vi "Close Connection.vi"(8 "error in (no error)":errorcluster, 11 "Connection Reference In":refnum<data-value>) -> (0 "error out":errorcluster)   [LabVIEW 2020, in "Connection Reference.lvlib" / "Connection Reference.lvclass"]
uses:
  <vilib>/gpm_packages/@cs/Network-interface/Source/Connection Reference/Connection Reference/Connection Reference.lvclass
  <vilib>/gpm_packages/@cs/Network-interface/Source/Connection Reference/Connection Reference/Connection Reference.lvclass/Connection Reference.ctl
  <vilib>/gpm_packages/@cs/Network-interface/Source/Connection Reference/IConnection/IConnection.lvclass
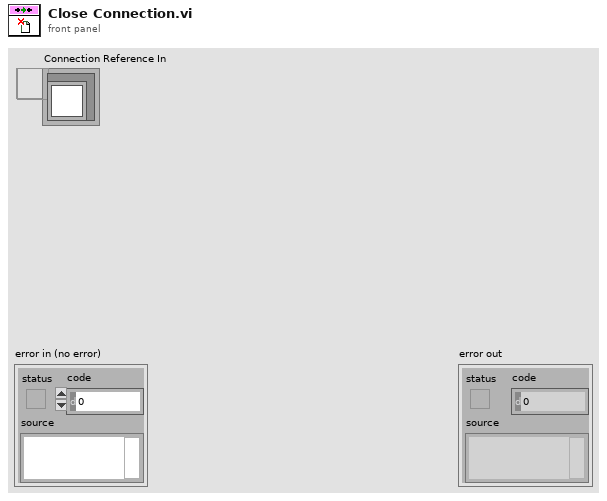
[diagram p1: front panel]
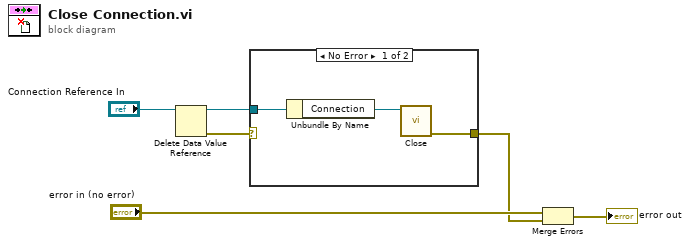
[diagram p0: block diagram]
diagram:
  n1 = Delete Data Value Reference(data value reference="Connection Reference In") -> (data value=w5:refnum<class "Connection Reference.lvclass">, error out=w4:errorcluster)  [unwired: 1 in]
  n2 = case shown="No Error" w4 {
    selector: w4 -> [_ w10]
    tunnel: w5 -> [w9 _]
    tunnel: [w7 w10] -> w2
    frame No Error {
      n3 = Unbundle By Name(w9) -> ("Connection"=w8:refnum<class "IConnection.lvclass">)
      n4 = call-dynamic "Close.vi"("IConnection in"=w8) -> ("error out"=w7:errorcluster)  [unwired: 10 in]
    }
    frame Error {
    }
  }
  n5 = Merge Errors("error in (no error)", w2) -> (→"error out":errorcluster)
